vi "Toggle Symbol.vi"(6 "Coords":T1, 11 "Display State In":T2) -> (3 "Display State In 2":T2 caption="Display State In")   [LabVIEW 2014]
uses:
  State ListBox.ctl
  <vilib>/Utility/miscctls.llb/LVPoint32TypeDef.ctl
  ListBox XControl.xctl
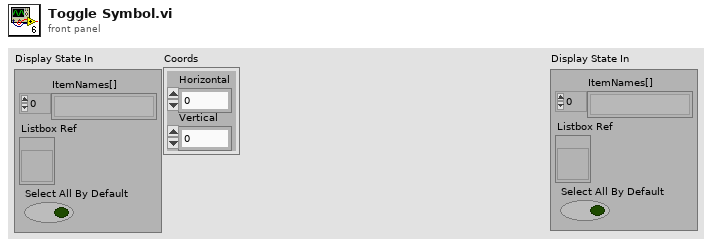
[diagram p1: front panel]
types:
  T1 = typedef "LVPoint32TypeDef.ctl" = cluster{"Horizontal":i32, "Vertical":i32}
  T2 = typedef "ListBox XControl.xctl/State ListBox.ctl" = cluster{"ItemNames[]":string[], "Listbox Ref":refnum<vi>, "Select All By Default":bool}
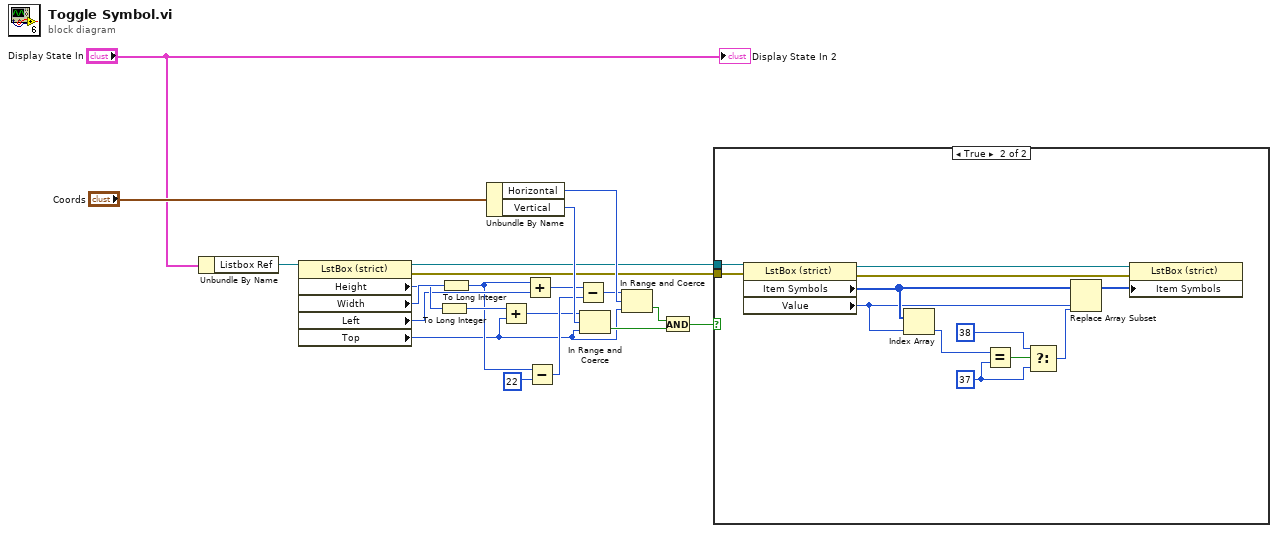
[diagram p0: block diagram]
diagram:
  n1 = Unbundle By Name("Display State In") -> ("Listbox Ref"=w5:refnum<vi>)
  n2 = property class="LstBox (strict)"(reference=w5) -> (reference out=w3:refnum<vi>, error out=w2:errorcluster, "Height"=w16:u32, "Width"=w17:u32, "Left"=w14:i32, "Top"=w4:i32)  [unwired: 1 in]
  n3 = To Long Integer(number=w16) -> (32bit integer=w15:i32)
  n4 = To Long Integer(number=w17) -> (32bit integer=w12:i32)
  n5 = Unbundle By Name("Coords") -> ("Horizontal"=w21:i32, "Vertical"=w20:i32)
  n6 = Add(x=w15, y=w4) -> (x+y=w8:i32)
  n7 = Add(x=w12, y=w14) -> (x+y=w13:i32)
  n8 = Subtract(x=w12, y=22) -> (x-y=w10:i32)
  n9 = Subtract(x=w13, y=w10) -> (x-y=w9:i32)
  n10 = In Range and Coerce(upper limit=w8, x=w20, lower limit=w4) -> (In Range?=w18:bool)  [unwired: 1 out]
  n11 = In Range and Coerce(upper limit=w9, x=w21, lower limit=w4) -> (In Range?=w19:bool)  [unwired: 1 out]
  n12 = And(x=w19, y=w18) -> (x .and. y?=w1:bool)
  n13 = case shown="True" w1 {
    tunnel: w3 -> [_ w23]
    tunnel: w2 -> [_ w22]
    frame False {
    }
    frame True {
      w30 = 37 ("y")
      n14 = property class="LstBox (strict)"(reference=w23, error in=w22) -> (reference out=w26:refnum<vi>, error out=w25:errorcluster, "Item Symbols"=w33:i32[], "Value"=w27:i32)
      n15 = Index Array(array=w33, index=w27) -> (element=w32:i32)
      n16 = Equal?(x=w32, y=w30) -> (x = y?=w31:bool)
      n17 = Select(t=38, s=w31, f=w30) -> (s? t:f=w28:i32)
      n18 = Replace Array Subset(array=w33, new element=w28, index=w27) -> (w24:i32[])
      n19 = property class="LstBox (strict)"(reference=w26, error in=w25, "Item Symbols"=w24) -> ()  [unwired: 2 out]
    }
  }
  "Display State In 2" <- "Display State In"
